vi "sensor averaging.vi"(0 "sensor chanel cluster":T1, 1 "array":dbl[](array[numeric]), 2 "array 2":dbl[](array[numeric]), 3 "array 3":dbl[](array[numeric]), 4 "array 4":dbl[](array[numeric]), 5 "array 5":dbl[](array[numeric]), 6 "avg win1":i32=24, 7 "avg win2":i32=24, 8 "array sensor in":dbl[](array[numeric]), 9 "error in":errorcluster, 11 "denois level array":dbl[](array[numeric])) -> (19 "error out":errorcluster, 21 "output array":dbl[](array[numeric]), 22 "output array 2":dbl[](array[numeric]), 23 "output array 3":dbl[](array[numeric]), 24 "output array 4":dbl[](array[numeric]), 25 "output array 5":dbl[](array[numeric]), 26 "avg data array":dbl[](array[numeric]), 27 "orgin data":dbl[](array[numeric]))   [LabVIEW 2019]
panel:
  out "element":dbl
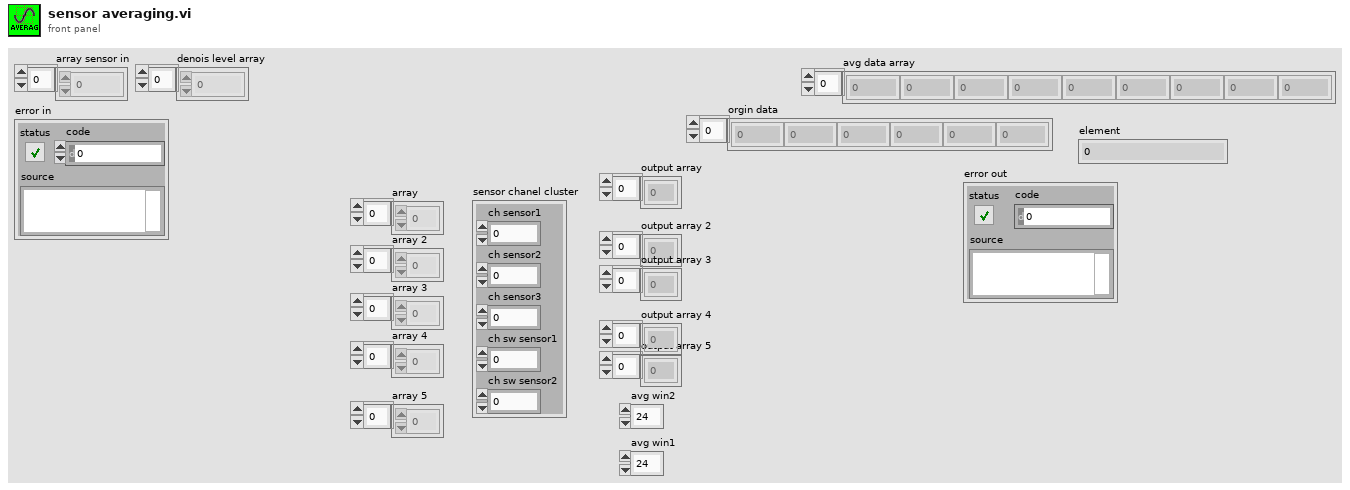
[diagram p1: front panel]
types:
  T1 = cluster{"ch sensor1":dbl, "ch sensor2":dbl, "ch sensor3":dbl, "ch sw sensor1":dbl, "ch sw sensor2":dbl}
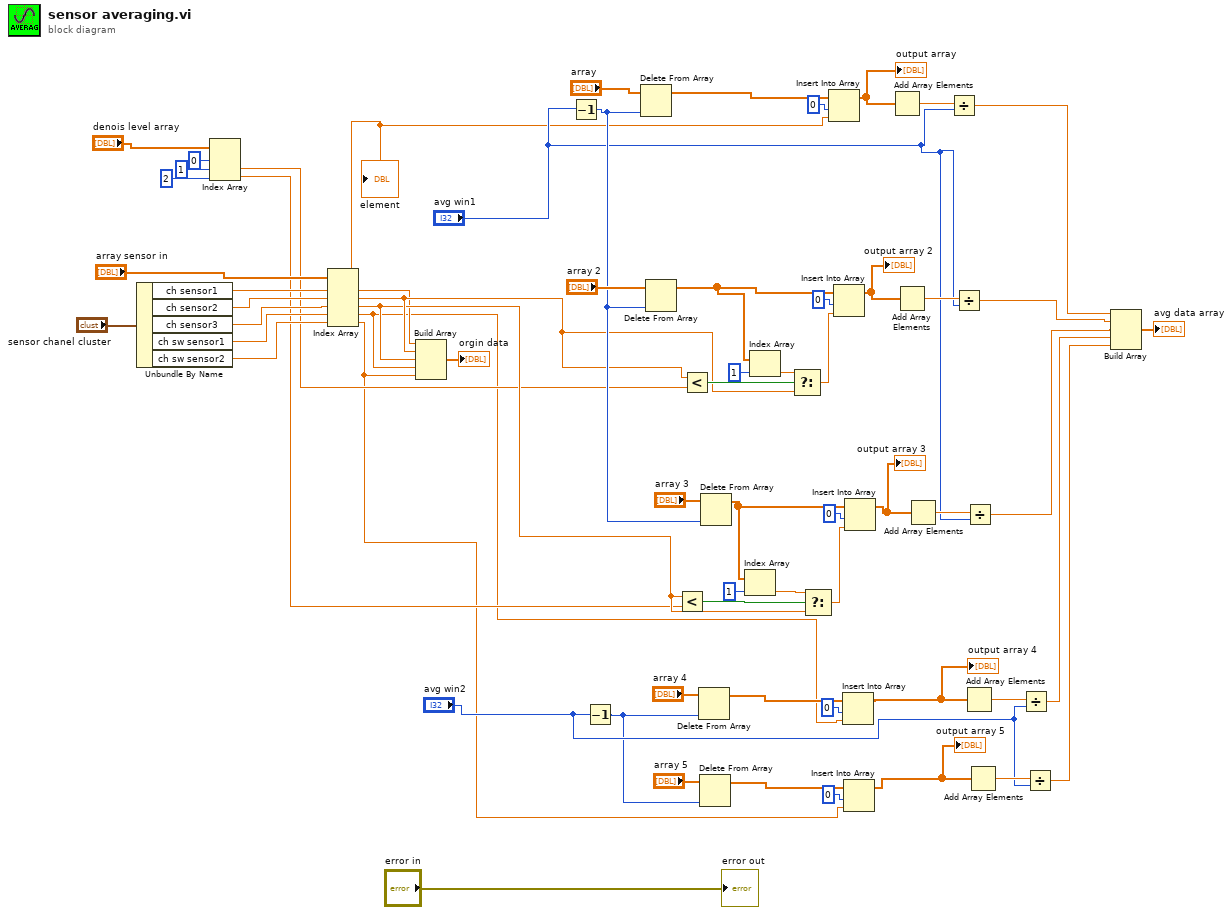
[diagram p0: block diagram]
diagram:
  n1 = Unbundle By Name("sensor chanel cluster") -> ("ch sensor1"=w40:dbl, "ch sensor2"=w39:dbl, "ch sensor3"=w38:dbl, "ch sw sensor1"=w37:dbl, "ch sw sensor2"=w36:dbl)
  n2 = Index Array(array="denois level array", index #1=0 ("index"), index #2=1 ("index"), index #3=2 ("index")) -> (element #2=w6:dbl, element #3=w5:dbl)  [unwired: 1 out]
  n3 = Index Array(array="array sensor in", index #1=w40, index #2=w39, index #3=w38, index #4=w37, index #5=w36) -> (element #1=w3:dbl, element #2=w20:dbl, element #3=w14:dbl, element #4=w1:dbl, element #5=w2:dbl)
  "element" <- w3
  n4 = Build Array(w3, w20, w14, w1, w2) -> (→"orgin data":dbl[])
  n5 = Decrement(x="avg win1") -> (x-1=w27:i32)
  n6 = Decrement(x="avg win2") -> (x-1=w4:i32)
  n7 = Delete From Array(array="array", index=w27) -> (array with subset deleted=w11:dbl[])  [unwired: 1 in, 1 out]
  n8 = Delete From Array(array="array 2", index=w27) -> (array with subset deleted=w21:dbl[])  [unwired: 1 in, 1 out]
  n9 = Less?(x=w14, y=w5) -> (x < y?=w18:bool)
  n10 = Less?(x=w20, y=w6) -> (x < y?=w22:bool)
  n11 = Delete From Array(array="array 4", index=w4) -> (array with subset deleted=w49:dbl[])  [unwired: 1 in, 1 out]
  n12 = Delete From Array(array="array 5", index=w4) -> (array with subset deleted=w46:dbl[])  [unwired: 1 in, 1 out]
  n13 = Delete From Array(array="array 3", index=w27) -> (array with subset deleted=w15:dbl[])  [unwired: 1 in, 1 out]
  n14 = Index Array(array=w15, index=1) -> (element=w16:dbl)
  n15 = Index Array(array=w21, index=1) -> (element=w24:dbl)
  n16 = Select(t=w24, s=w22, f=w20) -> (s? t:f=w19:dbl)
  n17 = Select(t=w16, s=w18, f=w14) -> (s? t:f=w13:dbl)
  n18 = Insert Into Array(array=w11, index=0, new element=w3) -> (w60:dbl[])
  "output array" <- w60
  n19 = Insert Into Array(array=w21, index=0, new element=w19) -> (w59:dbl[])
  "output array 2" <- w59
  n20 = Insert Into Array(array=w49, index=0, new element=w1) -> (w42:dbl[])
  "output array 4" <- w42
  n21 = Insert Into Array(array=w46, index=0, new element=w2) -> (w41:dbl[])
  "output array 5" <- w41
  n22 = Insert Into Array(array=w15, index=0, new element=w13) -> (w52:dbl[])
  "output array 3" <- w52
  n23 = Add Array Elements(numeric array=w60) -> (sum=w61:dbl)
  n24 = Add Array Elements(numeric array=w59) -> (sum=w58:dbl)
  n25 = Add Array Elements(numeric array=w52) -> (sum=w53:dbl)
  n26 = Divide(x=w61, y="avg win1") -> (x/y=w34:dbl)
  n27 = Divide(x=w58, y="avg win1") -> (x/y=w33:dbl)
  n28 = Add Array Elements(numeric array=w42) -> (sum=w43:dbl)
  n29 = Divide(x=w53, y="avg win1") -> (x/y=w32:dbl)
  n30 = Add Array Elements(numeric array=w41) -> (sum=w44:dbl)
  n31 = Divide(x=w43, y="avg win2") -> (x/y=w31:dbl)
  n32 = Divide(x=w44, y="avg win2") -> (x/y=w30:dbl)
  n33 = Build Array(w34, w33, w32, w31, w30) -> (→"avg data array":dbl[])
  "error out" <- "error in"
